vi "solar_voy_def Export (cmd_tlm_server).vi"(8 "error in (no error)":errorcluster, 10 "INTERFACES to Merge":T1[](array[typedef]), 11 "cmd_tlm_server.txt in":path) -> (0 "error out":errorcluster, 2 "Preview cmd_tlm_server":string, 3 "cmd_tlm_server.txt out":path)   [LabVIEW 2018]
doc: "This exports the COSMOS command and telemetry server file to the corresponding COSMOS configuration folder:\ncosmos\\config\\targets\\TARGET\\cmd_tlm_server.txt"
uses:
  solar_voy_def_ctl INTERFACE.ctl
panel:
  in  "Suppress Errors? (T)":bool=TRUE
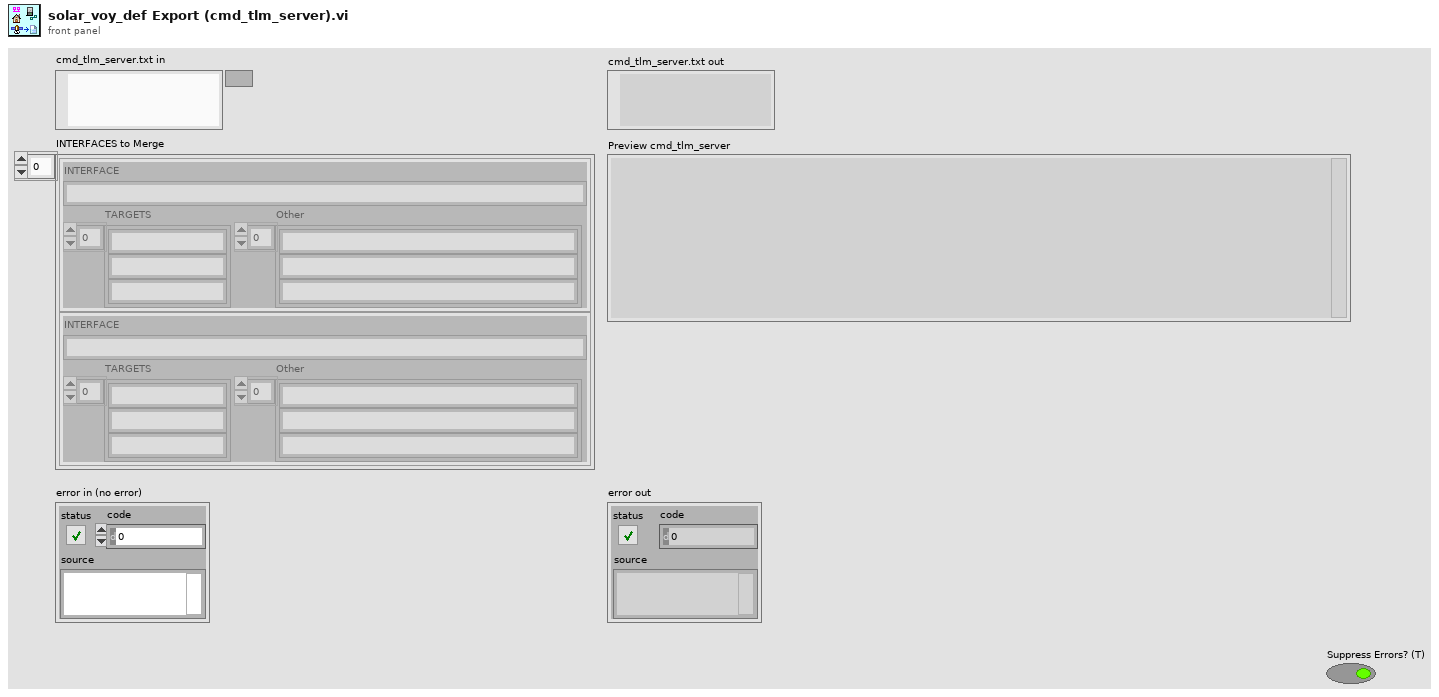
[diagram p1: front panel]
types:
  T1 = typedef "solar_voy_def_ctl INTERFACE.ctl" = cluster{"INTERFACE":string, "TARGETS":string[], "Other":string[]}
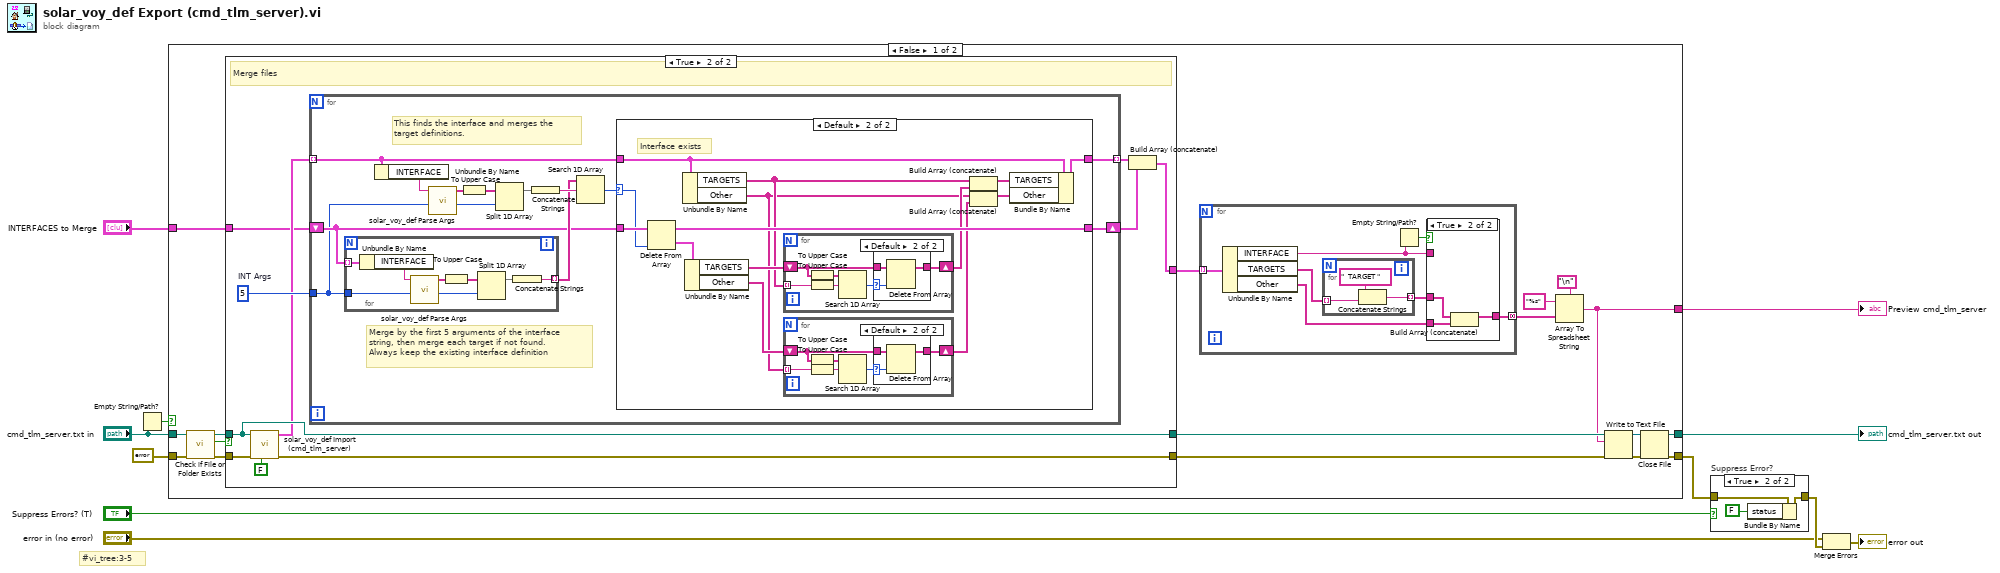
[diagram p0: block diagram]
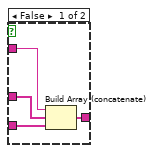
[diagram p6: hidden frame]
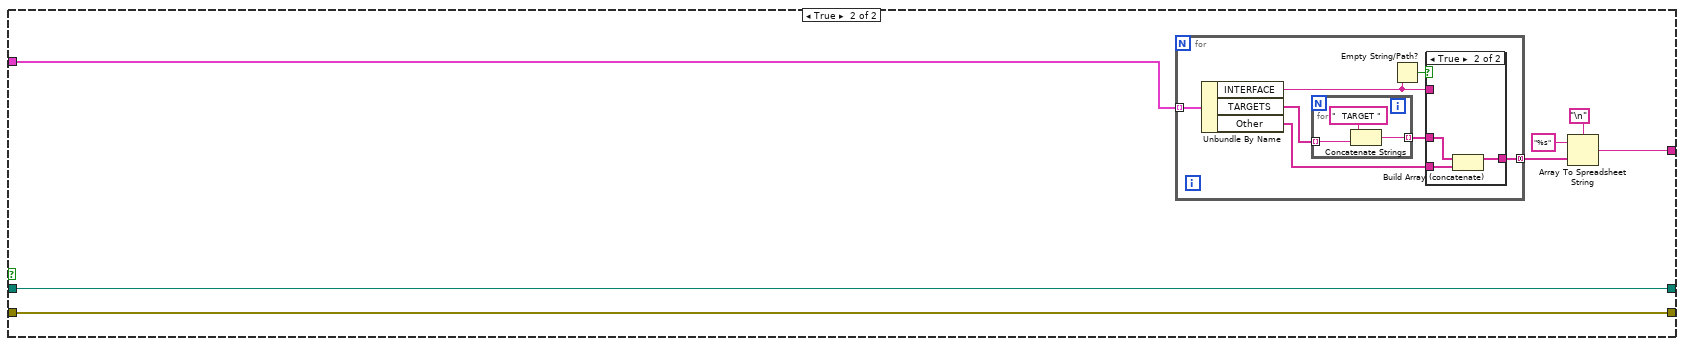
[diagram p7: hidden frame]
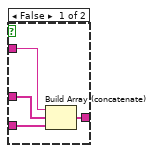
[diagram p8: hidden frame]
diagram:
  # "#vi_tree:3-5"
  n1 = Empty String/Path?(string/path="cmd_tlm_server.txt in") -> (empty?=w11:bool)
  n2 = case shown="False" w11 {
    tunnel: errorcluster {"status"=FALSE, "code"=0, "source"=""} ("error in (no error)") -> [w24 w120]
    tunnel: [w26 w120] -> w4
    tunnel: "cmd_tlm_server.txt in" -> [w14 w119]
    tunnel: [w25 w119] -> w8
    tunnel: "INTERFACES to Merge" -> [w16 w115]
    tunnel: [w15 w114] -> w10
    frame False {
      n3 = call <vilib>:"Check if File or Folder Exists.vi"("error in (no error)"=w24, "path"=w14) -> ("error out"=w21:errorcluster, "file or folder exists?"=w19:bool, "dup path"=w20:path)  [unwired: 7 in]
      n4 = case shown="True" w19 {
        tunnel: [w30 w40] -> w23
        tunnel: [w31 w39] -> w22
        tunnel: w21 -> [w30 w41]
        tunnel: w20 -> [w31 w39]
        tunnel: w16 -> [w29 w34]
        tunnel: [w29 w33] -> w13
        frame False {
          # "File not found"
        }
        frame True {
          w38 = 5  # INT Args
          # "Merge files"
          n5 = call "solar_voy_def Import (cmd_tlm_server).vi"("Suppress Errors? (T)"=FALSE, "error in (no error)"=w41, "cmd_tlm_server.txt"=w39) -> ("error out"=w40:errorcluster, "INTERFACES"=w35:T1[])  [unwired: 7 in]
          n6 = for {
            tunnel: w35 -> [w47] mode=indexing
            tunnel: w38 -> [w42]
            shift-right: [w45] -> w36
            shift-left: w34 -> [w44]
            tunnel: [w43] -> w37 mode=indexing
            # "Merge by the first 5 arguments of the interface\nstring, then merge each target if not found.\nAlways keep the existing interface definition"
            # "This finds the interface and merges the\ntarget definitions."
            n7 = for {
              tunnel: w44 -> [w58] mode=indexing
              tunnel: [w55] -> w46 mode=indexing
              tunnel: w42 -> [w54]
              n8 = Unbundle By Name(w58) -> ("INTERFACE"=w60:string)
              n9 = call "solar_voy_def Parse Args.vi"("String"=w60) -> ("Arguments"=w59:string[])  [unwired: 10 in]
              n10 = To Upper Case(1:w59) -> (0:w57:string[])
              n11 = Split 1D Array(array=w57, index=w54) -> (first subarray=w56:string[])  [unwired: 1 out]
              n12 = Concatenate Strings(w56) -> (w55:string)
            }
            n13 = Unbundle By Name(w47) -> ("INTERFACE"=w50:string)
            n14 = call "solar_voy_def Parse Args.vi"("String"=w50) -> ("Arguments"=w51:string[])  [unwired: 10 in]
            n15 = To Upper Case(1:w51) -> (0:w52:string[])
            n16 = Split 1D Array(array=w52, index=w42) -> (first subarray=w53:string[])  [unwired: 1 out]
            n17 = Concatenate Strings(w53) -> (w49:string)
            n18 = Search 1D Array(1D array=w46, element=w49) -> (index of element=w48:i32)  [unwired: 1 in]
            n19 = case shown="Default" w48 {
              selector: w48 -> [_ w75]
              tunnel: w47 -> [w62 w72]
              tunnel: [w61 w74] -> w45
              tunnel: w44 -> [w61 w76]
              tunnel: [w62 w71] -> w43
              frame -1 {
                # "Interface not found"
              }
              frame Default {
                # "Interface exists"
                n20 = Delete From Array(array=w76, index=w75) -> (deleted portion=w73:T1, array with subset deleted=w74:T1[])  [unwired: 1 in]
                n21 = Unbundle By Name(w72) -> ("TARGETS"=w67:string[], "Other"=w63:string[])
                n22 = Unbundle By Name(w73) -> ("TARGETS"=w68:string[], "Other"=w66:string[])
                n23 = for {
                  tunnel: w67 -> [w92] mode=indexing
                  shift-right: [w89] -> w69
                  shift-left: w68 -> [w90]
                  n24 = To Upper Case(1:w90) -> (0:w88:string[])
                  n25 = To Upper Case(1:w92) -> (0:w87:string)
                  n26 = Search 1D Array(1D array=w88, element=w87) -> (index of element=w91:i32)  [unwired: 1 in]
                  n27 = case shown="Default" w91 {
                    selector: w91 -> [_ w95]
                    tunnel: w90 -> [w93 w96]
                    tunnel: [w93 w94] -> w89
                    frame -1 {
                    }
                    frame Default {
                      n28 = Delete From Array(array=w96, index=w95) -> (array with subset deleted=w94:string[])  [unwired: 1 in, 1 out]
                    }
                  }
                }
                n29 = for {
                  tunnel: w63 -> [w82] mode=indexing
                  shift-right: [w79] -> w65
                  shift-left: w66 -> [w80]
                  n30 = To Upper Case(1:w80) -> (0:w78:string[])
                  n31 = To Upper Case(1:w82) -> (0:w77:string)
                  n32 = Search 1D Array(1D array=w78, element=w77) -> (index of element=w81:i32)  [unwired: 1 in]
                  n33 = case shown="Default" w81 {
                    selector: w81 -> [_ w85]
                    tunnel: w80 -> [w83 w86]
                    tunnel: [w83 w84] -> w79
                    frame -1 {
                    }
                    frame Default {
                      n34 = Delete From Array(array=w86, index=w85) -> (array with subset deleted=w84:string[])  [unwired: 1 in, 1 out]
                    }
                  }
                }
                n35 = Build Array (concatenate)(w67, w69) -> (w70:string[])
                n36 = Build Array (concatenate)(w63, w65) -> (w64:string[])
                n37 = Bundle By Name(cluster=w72, "TARGETS"=w70, "Other"=w64) -> (w71:T1)
              }
            }
          }
          n38 = Build Array (concatenate)(w37, w36) -> (w33:T1[])
        }
      }
      n39 = for {
        tunnel: w13 -> [w103] mode=indexing
        tunnel: [w97] -> w12 mode=concatenating
        n40 = Unbundle By Name(w103) -> ("INTERFACE"=w99:string, "TARGETS"=w102:string[], "Other"=w100:string[])
        n41 = for {
          tunnel: w102 -> [w113] mode=indexing
          tunnel: [w111] -> w101 mode=indexing
          n42 = Concatenate Strings("  TARGET ", w113) -> (w111:string)
        }
        n43 = Empty String/Path?(string/path=w99) -> (empty?=w98:bool)
        n44 = case shown="True" w98 {
          tunnel: w101 -> [w107 w110]
          tunnel: w100 -> [w106 w109]
          tunnel: w99 -> [w105 _]
          tunnel: [w104 w108] -> w97
          frame False {
            n45 = Build Array (concatenate)(w105, w107, w106) -> (w104:string[])
          }
          frame True {
            n46 = Build Array (concatenate)(w110, w109) -> (w108:string[])
          }
        }
      }
      n47 = Array To Spreadsheet String(delimiter (Tab)="\n", array=w12, 3:"%s" ("format string")) -> (spreadsheet string=w15:string)
      n48 = Write to Text File(file (use dialog)=w22, text=w15, error in=w23) -> (refnum out=w27:refnum<file>, error out=w28:errorcluster)  [unwired: 1 in, 1 out]
      n49 = Close File(refnum=w27, error in=w28) -> (path=w25:path, error out=w26:errorcluster)
    }
    frame True {
      n50 = for {
        tunnel: w115 -> [w127] mode=indexing
        tunnel: [w121] -> w116 mode=concatenating
        n51 = Unbundle By Name(w127) -> ("INTERFACE"=w123:string, "TARGETS"=w126:string[], "Other"=w124:string[])
        n52 = for {
          tunnel: w126 -> [w137] mode=indexing
          tunnel: [w135] -> w125 mode=indexing
          n53 = Concatenate Strings("  TARGET ", w137) -> (w135:string)
        }
        n54 = Empty String/Path?(string/path=w123) -> (empty?=w122:bool)
        n55 = case shown="True" w122 {
          tunnel: w125 -> [w131 w134]
          tunnel: w124 -> [w130 w133]
          tunnel: w123 -> [w129 _]
          tunnel: [w128 w132] -> w121
          frame False {
            n56 = Build Array (concatenate)(w129, w131, w130) -> (w128:string[])
          }
          frame True {
            n57 = Build Array (concatenate)(w134, w133) -> (w132:string[])
          }
        }
      }
      n58 = Array To Spreadsheet String(delimiter (Tab)="\n" ("Line Feed Constant"), array=w116, 3:"%s" ("format string")) -> (spreadsheet string=w114:string)
    }
  }
  "Preview cmd_tlm_server" <- w10
  "cmd_tlm_server.txt out" <- w8
  n59 = case "Suppress Error?" shown="True" "Suppress Errors? (T)" {
    tunnel: w4 -> [w138 w141]
    tunnel: [w138 w140] -> w6
    frame False {
    }
    frame True {
      n60 = Bundle By Name(cluster=w141, "status"=FALSE) -> (w140:errorcluster)
    }
  }
  n61 = Merge Errors("error in (no error)", w6) -> (→"error out":errorcluster)
